vi "Follow Peaks.vi"(5 "Best fit guess":dbl[][](array[numeric]) format="%#_4p", 6 "Good fit?":dbl[](array[numeric]) format="%#_4p", 7 "Best fit results":dbl[][](array[numeric]) format="%#_4p", 8 "error in (no error)":errorcluster, 11 "Resonance Detector in":refnum<class "Resonance Detector.lvclass">) -> (0 "error out":errorcluster, 3 "Resonance Detector out":refnum<class "Resonance Detector.lvclass">)   [LabVIEW 2016, in "Resonance Detector.lvclass"]
uses:
  Resonance Detector.lvclass
  Spectrum Recorder too Messages/Update Focus Msg/Update Focus Msg.lvclass
  C:/Program Files/National Instruments/LabVIEW 2016/vi.lib/ActorFramework/Message/Message.lvclass
  Spectrum Recorder too Messages/Update Focus Msg/Update Focus Msg.lvclass/Update Focus Msg.ctl
  Spectrum Recorder too Messages/Update Focus Msg/Write Focus region centers.vi
  Read Line detector configuration.vi
panel:
  # "F0         dF     Ampl   Phase   Xbgrd   Ybgrd"
  # "F0         dF     Ampl   Phase   Xbgrd   Ybgrd    mask"
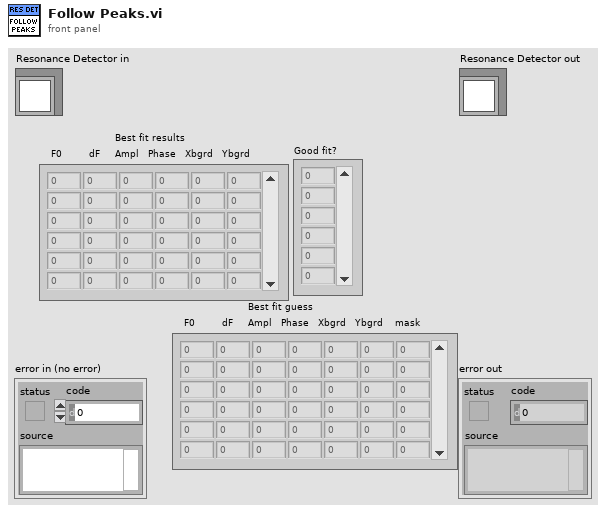
[diagram p1: front panel]
types:
  T1 = typedef "Line Detector Configuration.ctl" = cluster{"Peak width guess":dbl, "Background removal":enum16{"NONE", "High-pass", "Detrend"}, "Smoothing":enum16{"NONE", "Low-pass", "Denoise"}, "Smooth window":dbl, "Relative threshold":dbl, "Finder algorithm":enum16{"Basic", "Wavelet", "Wavelet+detrend"}, "Bgd window":dbl, "Spectrum recorder module name":string, "Fit window":dbl, "Initial fit guess":enum16{"Peak finder", "Last fit"}, "Follow\npeaks":bool, "Re-sample":dbl}
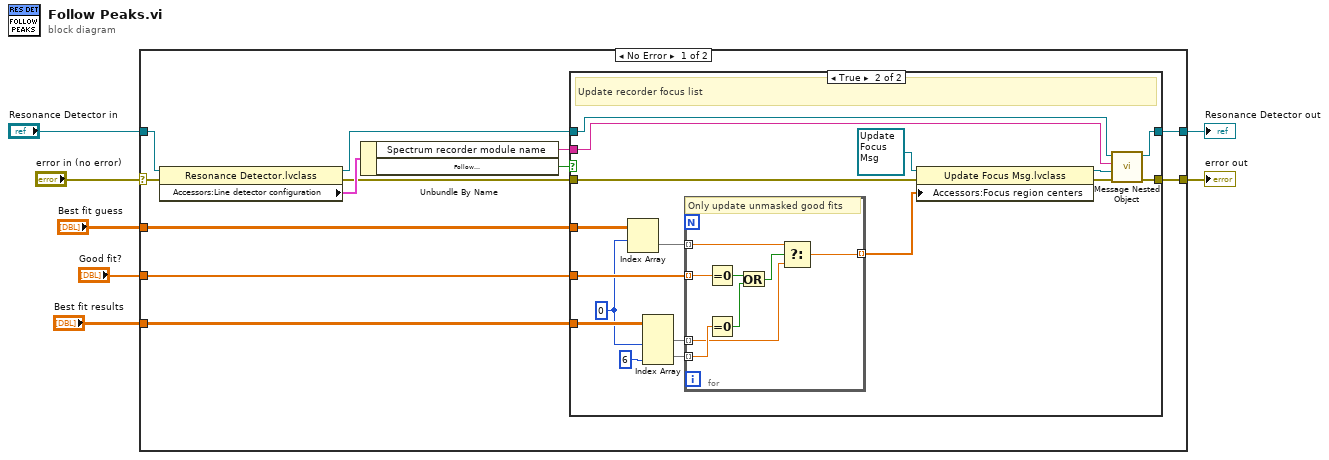
[diagram p0: block diagram]
diagram:
  n1 = case shown="No Error" "error in (no error)" {
    selector: "error in (no error)" -> [w11 w48]
    tunnel: [w12 w48] -> w6
    tunnel: [w13 w47] -> w4
    tunnel: "Resonance Detector in" -> [w9 w47]
    tunnel: "Best fit results" -> [w17 _]
    tunnel: "Good fit?" -> [w15 _]
    tunnel: "Best fit guess" -> [w10 _]
    frame No Error {
      n2 = property class="Resonance Detector.lvclass"(reference=w9, error in=w11) -> (reference out=w8:refnum<class "Resonance Detector.lvclass">, error out=w16:errorcluster, "Accessors:Line detector configuration"=w19:T1)
      n3 = Unbundle By Name(w19) -> ("Spectrum recorder module name"=w14:string, "Follow\npeaks"=w18:bool)
      n4 = case shown="True" w18 {
        tunnel: w16 -> [w20 w32]
        tunnel: [w20 w38] -> w12
        tunnel: [w21 w37] -> w13
        tunnel: w8 -> [w21 w36]
        tunnel: w17 -> [_ w35]
        tunnel: w14 -> [_ w34]
        tunnel: w15 -> [_ w28]
        tunnel: w10 -> [_ w24]
        frame False {
        }
        frame True {
          w23 = 0 ("index")
          # "Update recorder focus list"
          n5 = Index Array(array=w24, index (row)=w23) -> (element=w22:dbl[])  [unwired: 1 in]
          n6 = Index Array(array=w35, index (col) #1=w23, index (col) #2=6 ("index (col)")) -> (element #1=w27:dbl[], element #2=w26:dbl[])  [unwired: 2 in]
          n7 = for {
            tunnel: w28 -> [w46] mode=indexing
            tunnel: w27 -> [w41] mode=indexing
            tunnel: w26 -> [w44] mode=indexing
            tunnel: [w40] -> w25 mode=indexing
            tunnel: w22 -> [w39] mode=indexing
            # "Only update unmasked good fits"
            n8 = Equal To 0?(x=w46) -> (x = 0?=w45:bool)
            n9 = Equal To 0?(x=w44) -> (x = 0?=w43:bool)
            n10 = Or(x=w45, y=w43) -> (x .or. y?=w42:bool)
            n11 = Select(t=w39, s=w42, f=w41) -> (s? t:f=w40:dbl)
          }
          n12 = property class="Update Focus Msg.lvclass"(reference=refnum<class "Update Focus Msg.lvclass"> refnum ("Update Focus Msg.lvclass"), error in=w32, "Accessors:Focus region centers"=w25) -> (reference out=w31:refnum<class "Update Focus Msg.lvclass">, error out=w30:errorcluster)
          n13 = call-dynamic "Message Nested Object.vi"("error in (no error)"=w30, "Message"=w31, "Name"=w34, "Application Controller in"=w36) -> ("error out"=w38:errorcluster, "Application Controller out"=w37:refnum<class "Resonance Detector.lvclass">)  [unwired: 6 in]
        }
      }
    }
    frame Error {
    }
  }
  "error out" <- w6
  "Resonance Detector out" <- w4
